vi "Inst.Xeryon-Rotator.Set Angle.vi"(8 "error in (no error)":errorcluster, 10 "Angle (°)":dbl, 11 "Inst.Xeryon-Rotator in":refnum<class "Inst.Xeryon-Rotator.lvclass">) -> (0 "error out":errorcluster, 3 "Inst.Xeryon-Rotator out":refnum<class "Inst.Xeryon-Rotator.lvclass">)   [LabVIEW 2019, in "Inst.Xeryon-Rotator.lvclass"]
uses:
  Inst.Xeryon-Rotator.lvclass
  Inst.Xeryon-Rotator.lvclass/Inst.Xeryon-Rotator.ctl
  Controller.LV/Controller.LV.lvclass
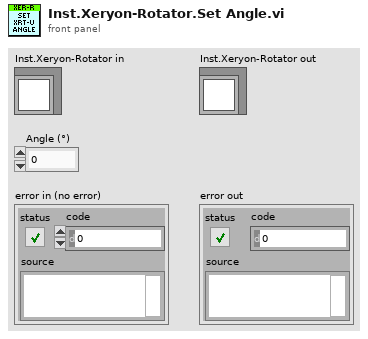
[diagram p1: front panel]
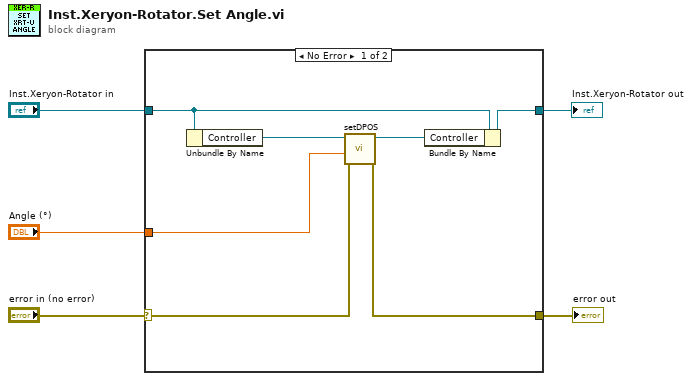
[diagram p0: block diagram]
diagram:
  n1 = case shown="No Error" "error in (no error)" {
    selector: "error in (no error)" -> [w7 w14]
    tunnel: [w12 w13] -> w5
    tunnel: "Inst.Xeryon-Rotator in" -> [w11 w13]
    tunnel: "Angle (°)" -> [w8 _]
    tunnel: [w6 w14] -> w1
    frame No Error {
      n2 = Unbundle By Name(w11) -> ("Controller"=w9:refnum<class "Controller.LV.lvclass">)
      n3 = call-dynamic "setDPOS.vi"("error in (no error)"=w7, "DPOS In Current Units"=w8, "Controller in"=w9) -> ("error out"=w6:errorcluster, "Controller out"=w10:refnum<class "Controller.LV.lvclass">)  [unwired: 7 in]
      n4 = Bundle By Name(cluster=w11, "Controller"=w10) -> (w12:refnum<class "Inst.Xeryon-Rotator.lvclass">)
    }
    frame Error {
    }
  }
  "error out" <- w1
  "Inst.Xeryon-Rotator out" <- w5
